vi "_UnitTest.ClusterToArray.vi"() -> ()   [LabVIEW 2017]
uses:
  File/_FileName Rule.ctl
  Data/_support/Get DataType Description String.vi
panel:
  out "String":string
  out "Cluster 2":variant
  out "Array 2":variant[](array[variant])
  out "Cluster":variant
  out "Array":variant[](array[variant])
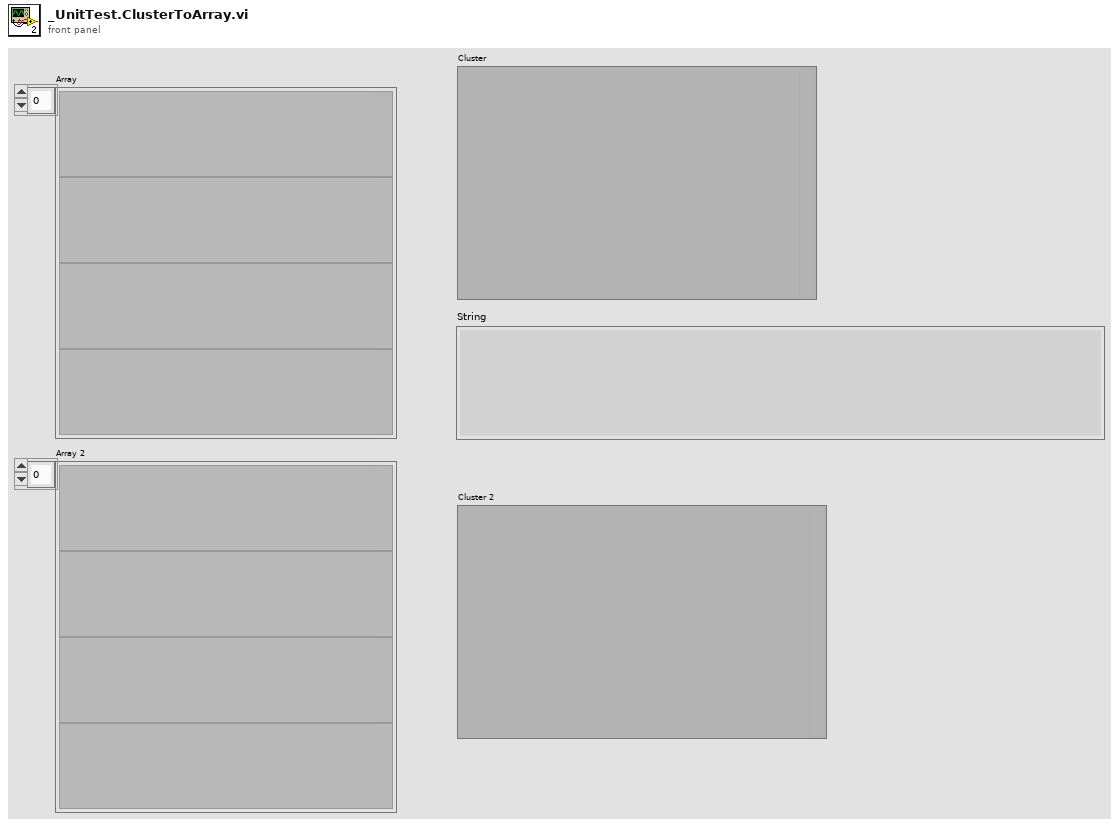
[diagram p1: front panel]
types:
  T1 = typedef "_FileName Rule.ctl" = cluster{"Rule":enum16{"Fixed File Name", "Indexed File Name", "TimeBased File Name"}, "Path":path, "filename":string}
  T2 = cluster{"status":bool, "code":i32, "source":string, "FileNameRule":T1}
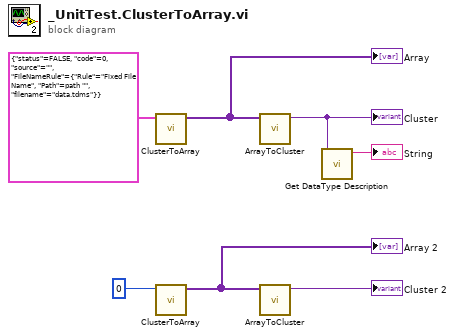
[diagram p0: block diagram]
diagram:
  n1 = call "ClusterToArray.vi"("Cluster"=T2 {"status"=FALSE, "code"=0, "source"="", "FileNameRule"={"Rule"=enum."Fixed File Name", "Path"=path "", "filename"="data.tdms"}} ("error in (no error)")) -> ("Array"=w6:variant[])  [unwired: 9 in, 1 out]
  "Array" <- w6
  n2 = call "ClusterToArray.vi"("Cluster"=0 ("code")) -> ("Array"=w4:variant[])  [unwired: 9 in, 1 out]
  "Array 2" <- w4
  n3 = call "ArrayToCluster.vi"("Array"=w6) -> ("Cluster"=w2:variant)  [unwired: 9 in, 1 out]
  "Cluster" <- w2
  n4 = call "ArrayToCluster.vi"("Array"=w4) -> ("Cluster"=→"Cluster 2":variant)  [unwired: 9 in, 1 out]
  n5 = call-poly "Get DataType Description.vi"("Variant"=w2) -> ("String"=→"String":string)  [unwired: 9 in, 1 out]
